vi "Shift Tab.vi"(8 "error in (no error)":errorcluster) -> (0 "error out":errorcluster)   [LabVIEW 2015, in "LVJSON.lvlib" / "Shared.lvlib"]
uses:
  Shared.lvlib
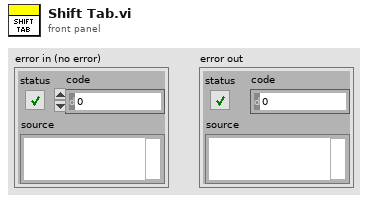
[diagram p1: front panel]
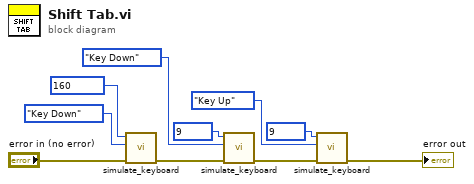
[diagram p0: block diagram]
diagram:
  n1 = call "simulate_keyboard.vi"("error in (no error)"="error in (no error)", "Direction"=enum16{"Key Down", "Key Up"}."Key Down", "Virtual Key"=u8 160) -> ("error out"=w3:errorcluster)  [unwired: 7 in]
  n2 = call "simulate_keyboard.vi"("error in (no error)"=w3, "Direction"=enum16{"Key Down", "Key Up"}."Key Down", "Virtual Key"=u8 9) -> ("error out"=w10:errorcluster)  [unwired: 7 in]
  n3 = call "simulate_keyboard.vi"("error in (no error)"=w10, "Direction"=enum16{"Key Down", "Key Up"}."Key Up", "Virtual Key"=u8 9) -> ("error out"=→"error out":errorcluster)  [unwired: 7 in]
